vi "Write Log Line.vi"(10 "log line":string, 11 "file handler in":refnum<class "File Handler.lvclass">) -> (0 "error out":errorcluster, 3 "file handler out":refnum<class "File Handler.lvclass">)   [LabVIEW 2018, in "GLog.lvlib" / "File Handler.lvclass"]
uses:
  File Handler.lvclass
  File Handler.lvclass/File Handler.ctl
  RolloverTrigger/RolloverTrigger.lvclass
panel:
  # "Connector Pane"
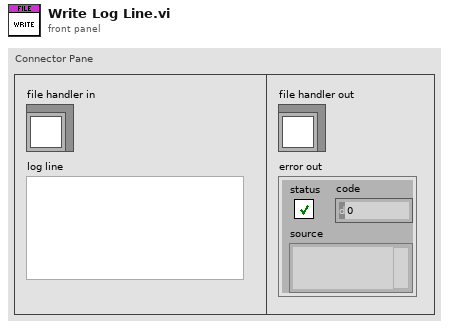
[diagram p1: front panel]
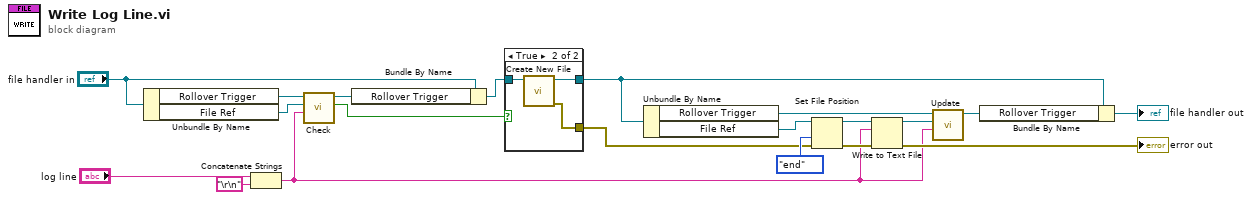
[diagram p0: block diagram]
diagram:
  n1 = Unbundle By Name("file handler in") -> ("Rollover Trigger"=w14:refnum<class "RolloverTrigger.lvclass">, "File Ref"=w10:refnum<file>)
  n2 = Concatenate Strings("log line", "\r\n") -> (w8:string)
  n3 = call-dynamic "Check.vi"("log line"=w8, "current file"=w10, "RolloverTrigger in"=w14) -> ("rollover?"=w13:bool, "RolloverTrigger out"=w11:refnum<class "RolloverTrigger.lvclass">)  [unwired: 7 in]
  n4 = Bundle By Name(cluster="file handler in", "Rollover Trigger"=w11) -> (w12:refnum<class "File Handler.lvclass">)
  n5 = case shown="True" w13 {
    tunnel: w12 -> [w21 w24]
    tunnel: [_ w22] -> w17
    tunnel: [w21 w23] -> w5
    frame False {
    }
    frame True {
      n6 = call "Create New File.vi"("file handler in"=w24) -> ("error out"=w22:errorcluster, "file handler out"=w23:refnum<class "File Handler.lvclass">)  [unwired: 9 in]
    }
  }
  n7 = Unbundle By Name(w5) -> ("Rollover Trigger"=w2:refnum<class "RolloverTrigger.lvclass">, "File Ref"=w3:refnum<file>)
  n8 = Set File Position(refnum=w3, from (0:start)=enum16{"start", "end", "current"}."end", error in=w17) -> (refnum out=w7:refnum<file>, error out=w20:errorcluster)  [unwired: 1 in]
  n9 = Write to Text File(file (use dialog)=w7, text=w8, error in=w20) -> (refnum out=w1:refnum<file>, error out=→"error out":errorcluster)  [unwired: 1 in, 1 out]
  n10 = call-dynamic "Update.vi"("log line"=w8, "file ref"=w1, "rollover trigger in"=w2) -> ("rollover trigger out"=w6:refnum<class "RolloverTrigger.lvclass">)  [unwired: 8 in]
  n11 = Bundle By Name(cluster=w5, "Rollover Trigger"=w6) -> (→"file handler out":refnum<class "File Handler.lvclass">)
